vi "获取VI中指定条件的控件名称列表.vi"(5 "名称包含":string[](array[string]), 7 "类名(Digital)":string="Digital", 8 "错误输入（无错误）":errorcluster, 11 "路径":path) -> (0 "错误输出":errorcluster, 2 "名称列表":string[](array[string]), 3 "获取控件引用":refnum<vi>[](array[refnum]))   [LabVIEW 2018]
doc: "使用类名对选择VI中的控件进行分类，并输出指定的类名的控件标签文本。如果名称包含为空，则不对其进行筛选，如果包含字符串，则按照字符串内容对其进行筛选。"
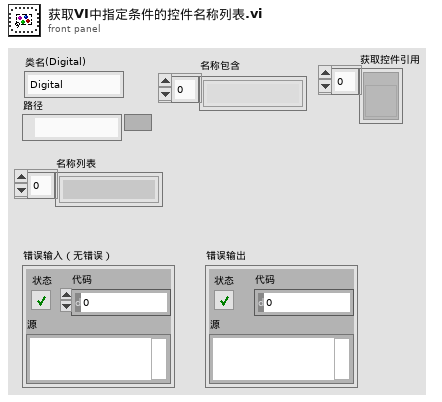
[diagram p1: front panel]
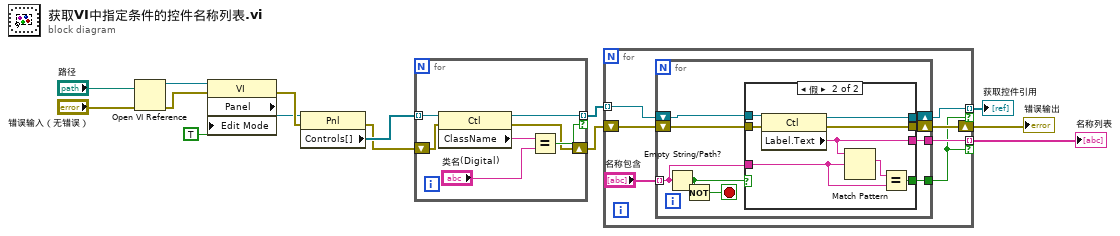
[diagram p0: block diagram]
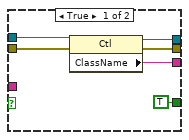
[diagram p2: hidden frame]
diagram:
  n1 = Open VI Reference(vi path="路径", error in (no error)="错误输入（无错误）") -> (vi reference=w9:refnum<vi>, error out=w10:errorcluster)  [unwired: 4 in]
  n2 = property class="VI"(reference=w9, error in=w10, "Edit Mode"=TRUE ("以编辑模式打开")) -> (error out=w13:errorcluster, "Panel"=w12:refnum<vi>)  [unwired: 1 out]
  n3 = property class="Pnl"(reference=w12, error in=w13) -> (error out=w6:errorcluster, "Controls[]"=w14:refnum<vi>[])  [unwired: 1 out]
  n4 = for {
    tunnel: w14 -> [w21] mode=indexing
    tunnel: [w19] -> w5 mode=indexing if=w18
    shift-right: [w15] -> w4
    shift-left: w6 -> [w16]
    n5 = property class="Ctl"(reference=w21, error in=w16) -> (reference out=w19:refnum<vi>, error out=w15:errorcluster, "ClassName"=w20:string)
    n6 = Equal?(x=w20, y="类名(Digital)") -> (x = y?=w18:bool)
  }
  n7 = for {
    tunnel: w5 -> [w28] mode=indexing
    tunnel: [w26] -> w2 mode=indexing if=w23
    shift-right: [w25] -> w3
    shift-left: w4 -> [w27]
    tunnel: [w24] -> w1 mode=indexing if=w23
    n8 = for {
      tunnel: [w35] -> w26
      tunnel: [w32] -> w23
      shift-right: [w33] -> w24
      shift-left: w28 -> [w37]
      shift-right: [w34] -> w25
      shift-left: w27 -> [w36]
      tunnel: "名称包含" -> [w31] mode=indexing
      stop <- w29 stop-if-true
      n9 = Empty String/Path?(string/path=w31) -> (empty?=w30:bool)
      n10 = Not(x=w30) -> (.not. x?=w29:bool)
      n11 = case shown="假" w30 {
        tunnel: w37 -> [w43 w51]
        tunnel: w36 -> [w42 w50]
        tunnel: [w41 w47] -> w35
        tunnel: [w40 w49] -> w34
        tunnel: [w39 w48] -> w33
        tunnel: w31 -> [_ w46]
        tunnel: [TRUE w44] -> w32
        frame True {
          n12 = property class="Ctl"(reference=w43, error in=w42) -> (reference out=w39:refnum<vi>, error out=w40:errorcluster, "ClassName"=w41:string)
        }
        frame False {
          n13 = property class="Ctl"(reference=w51, error in=w50) -> (reference out=w48:refnum<vi>, error out=w49:errorcluster, "Label.Text"=w47:string)
          n14 = Match Pattern(string=w47, regular expression=w46) -> (match substring=w45:string)  [unwired: 1 in, 3 out]
          n15 = Equal?(x=w45, y=w46) -> (x = y?=w44:bool)
        }
      }
    }
  }
  "错误输出" <- w3
  "名称列表" <- w2
  "获取控件引用" <- w1
